vi "Move Sciscan Scope.vi"(7 "Type":enum16{"Relative", "Absolute"}(ring)=enum."Absolute", 8 "error in":errorcluster, 10 "Displacement [um]":T1, 11 "GFG Refnum":refnum<vi>) -> (0 "error out":errorcluster, 3 "GFG Refnum Out":refnum<vi>)   [LabVIEW 2012, in "Sciscan Scope Daemon.lvlib"]
uses:
  Sciscan Scope Daemon.lvlib
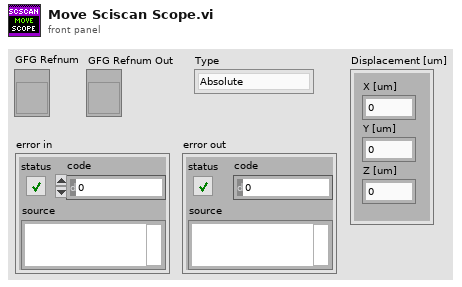
[diagram p1: front panel]
types:
  T1 = cluster{"X [um]":dbl, "Y [um]":dbl, "Z [um]":dbl}
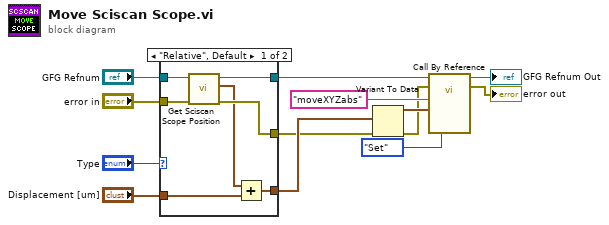
[diagram p0: block diagram]
diagram:
  n1 = case shown="\"Relative\", Default" "Type" {
    tunnel: "Displacement [um]" -> [w16 w23]
    tunnel: [w20 w23] -> w6
    tunnel: [w19 w22] -> w5
    tunnel: [w18 w21] -> w4
    tunnel: "GFG Refnum" -> [w15 w22]
    tunnel: "error in" -> [w14 w21]
    frame "Relative", Default {
      n2 = call "Get Sciscan Scope Position.vi"("error in"=w14, "GFG Refnum"=w15) -> ("error out"=w18:errorcluster, "Position [um]"=w17:T1, "GFG Refnum Out"=w19:refnum<vi>)  [unwired: 7 in]
      n3 = Add(x=w17, y=w16) -> (x+y=w20:T1)
    }
    frame "Absolute" {
    }
  }
  n4 = Variant To Data(error in=w4, type=w6, Variant=w6) -> (data=w7:T1, error out=w3:errorcluster)
  n5 = call-by-ref "?"(reference=w5, error in=w3, "Variable Name in"="moveXYZabs", "Variant in"=w7, "Action"=enum16{"Init", "Set", "Get"}."Set") -> (reference out=→"GFG Refnum Out":refnum<vi>, error out=→"error out":errorcluster)  [unwired: 10 in, 7 out]
